vi "get.p.vi"(0 "Session in":T1, 7 "error in":errorcluster) -> (20 "Image Out":T2, 22 "Session Out":T1, 27 "error out":errorcluster)   [LabVIEW 2017]
doc: "Creates, and edits acquisitions using the NI Vision Acquisition Express VI.\n\nThe NI Vision Acquisition Wizard is launched by placing the Express VI on the block diagram. Select an acquisition source and configure an acquisition using NI-IMAQ, NI-IMAQdx, or simulate an acquisition by reading an AVI or image files from a folder. After an acquisition is configured, select controls and indicators to be able to programmatically set in LabVIEW. Double-click the Vision Acquisition Express VI to edit the acquisition.\n\nNote: Any images created by the Express VI need to be disposed after use. Use the IMAQ Dispose.vi to cleanup the images output by the Express VI when they are no longer needed."
uses:
  <vilib>/vision/Image Controls.llb/IMAQ Image.ctl
  <vilib>/userdefined/High Color/IMAQdx.ctl
  <vilib>/vision/driver/NI_Vision_Acquisition_Software.lvlib
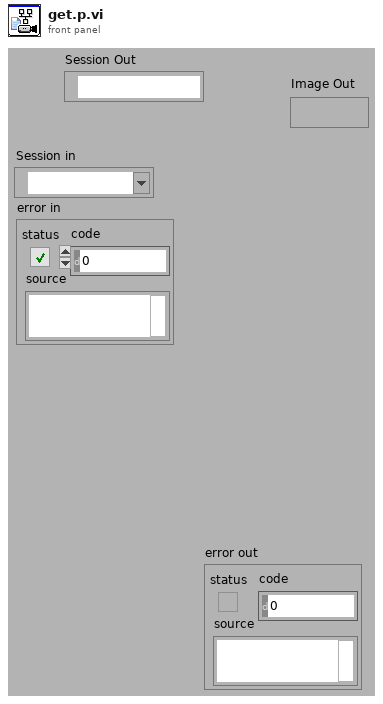
[diagram p1: front panel]
types:
  T1 = typedef "IMAQdx.ctl" = refnum<k21>
  T2 = typedef "IMAQ Image.ctl" = refnum<image>
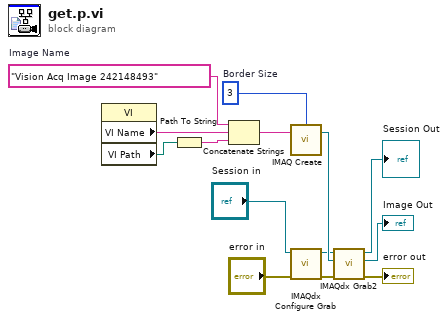
[diagram p0: block diagram]
diagram:
  w9 = 3  # Border Size
  w10 = "Vision Acq Image 242148493"  # Image Name
  n1 = property class="VI"() -> ("VI Name"=w13:string, "VI Path"=w14:path)  [unwired: 2 in, 2 out]
  n2 = Path To String(path=w14) -> (string=w12:string)
  n3 = Concatenate Strings(w10, w13, w12) -> (w11:string)
  n4 = call "IMAQ Create"("Border Size"=w9, "Image Name"=w11) -> ("New Image"=w8:T2)  [unwired: 2 in, 2 out]
  n5 = call <vilib>:"IMAQdx Configure Grab.vi"("error in"="error in", "Session In"="Session in") -> ("error out"=w6:errorcluster, "Session Out"=w7:T1)  [unwired: 8 in]
  n6 = call <vilib>:"IMAQdx Grab2.vi"("error in"=w6, "Image In"=w8, "Session In"=w7) -> ("error out"=→"error out":errorcluster, "Image Out"=→"Image Out":T2, "Session Out"=→"Session Out":T1)  [unwired: 5 in, 1 out]
